vi "MALT SplitList.vi"(3 "Line":string) -> (1 "Items":string[](array[string]))   [LabVIEW 2018, in "AltonTech MALT200817.lvlib"]
uses:
  AltonTech MALT200817.lvlib
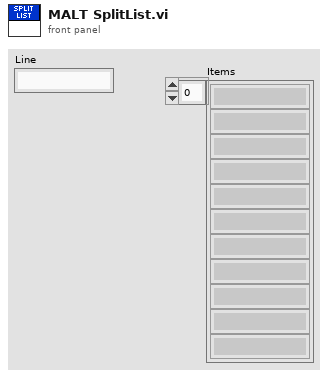
[diagram p1: front panel]
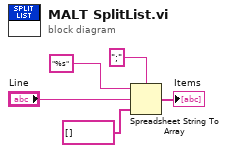
[diagram p0: block diagram]
diagram:
  n1 = Spreadsheet String To Array(delimiter (Tab)=";", format string="%s", spreadsheet string="Line", array type (2D Dbl)=string[] []) -> (array=→"Items":string[])
